vi "LabFrog2.vi"(8 "Simutation":bool, 11 "FROG path":path=path "C:/FROG") -> (0 "error out":errorcluster, 2 "ExpFrog":dbl[][][](array[numeric]), 3 "FROG data":T1[](array[typedef])=[{"Delay increment"=36.8, "Center Wavelength"=809.3, "Frog Error was"=0.0344, "Temporal FWHM"=100.0, "Spectral FWHM"=7.96, "FWHM Time-Bandwidth Product"=0.364, "RMS Time-Bandwidth Product"=0.85}, {"Delay increment"=36.8, "Center Wavelength"=809.3, "Frog Error was"=0.036, "Temporal FWHM"=98.9, "Spectral FWHM"=9.04, "FWHM Time-Bandwidth Product"=0.408, "RMS Time-Bandwidth Product"=0.858}])   [LabVIEW 2018]
doc: "LabFROG \n\nExtract data value from FROG file\n\nAndré Romero - 2022\nandretec@ifsc.usp.br"
uses:
  FROG.ctl
  <vilib>/Utility/file.llb/Read Delimited Spreadsheet (DBL).vi
  <vilib>/regexp/Match Regular Expression.xnode
panel:
  out "index":i32=13
  out "max value (ms)":u32=2
  out "Delay":u32[](array[numeric])=[0, 1, 1, 0, 1, 1, 1, 1, 0, 1, 0, 1, 0, 2, 0, 1, 0, 1, 1, 0, 1, 1, 0, 2, 1, 1, 1, 1, 1, 0, 1, 0, 1, 1, 1, 0, 1, 0, 1]
  out "FROG data":string[][](array[string])=[["32", "32"], ["36.8", "36.8"], ["809.3", "809.3"], ["0.0344", "0.036"], ["100", "98.9"], ["7.96", "9.04"], ["0.364", "0.408"], ["0.85", "0.858"], ["", ""]]
  out "FROG text data":string="Grid characteristics were: 32 points; Delay increment: 36.8 fs; Center Wavelength: 809.3 nm\nFrog Error was: 0.036\nTemporal FWHM: 98.9 fs\nSpectral FWHM: 9.04 nm\nFWHM Time-Bandwidth Product: 0.408\nRMS Time-Bandwidth Product: 0.858\n"
  out "filenames":string[](array[string])=["2022-05-26_10-35-10_ESpectral.dat", "2022-05-26_10-35-10_ETemporal.dat", "2022-05-26_10-35-10_ExpFrog.bmp", "2022-05-26_10-35-10_ExpFrog.dat", "2022-05-26_10-35-10_ExpFrog.jpg", "2022-05-26_10-35-10_Frog.dat", "2022-05-26_10-35-10_RawData.bmp", "2022-05-26_10-35-10_RawData.dat", "2022-05-26_10-35-10_RawData.jpg", "2022-05-26_10-35-10_RawData.png", "2022-05-26_10-35-10_RetrFrog.bmp", "2022-05-26_10-35-10_RetrFrog.dat", "2022-05-26_10-35-10_RetrFrog.jpg", "2022-05-26_10-35-10_screenShot.bmp", "2022-05-26_10-35-10_ss-colorpanel.jpg", "2022-05-26_10-35-10_ss-exper.jpg", "2022-05-26_10-35-10_ss-retrieved.jpg", "2022-05-26_10-35-10_ss-spectral.jpg", "2022-05-26_10-35-10_ss-temporal.jpg", "2022-05-26_10-35-16_ESpectral.dat", "2022-05-26_10-35-16_ETemporal.dat", "2022-05-26_10-35-16_ExpFrog.bmp", "2022-05-26_10-35-16_ExpFrog.dat", "2022-05-26_10-35-16_ExpFrog.jpg", "2022-05-26_10-35-16_Frog.dat", "2022-05-26_10-35-16_RawData.bmp", "2022-05-26_10-35-16_RawData.dat", "2022-05-26_10-35-16_RawData.jpg", "2022-05-26_10-35-16_RawData.png", "2022-05-26_10-35-16_RetrFrog.bmp", "2022-05-26_10-35-16_RetrFrog.dat", "2022-05-26_10-35-16_RetrFrog.jpg", "2022-05-26_10-35-16_screenShot.bmp", "2022-05-26_10-35-16_ss-colorpanel.jpg", "2022-05-26_10-35-16_ss-exper.jpg", "2022-05-26_10-35-16_ss-retrieved.jpg", "2022-05-26_10-35-16_ss-spectral.jpg", "2022-05-26_10-35-16_ss-temporal.jpg", "Thumbs.db"]
  # "[1] Delay increment"
  # "[2] Center Wavelength"
  # "[3] Frog Error was"
  # "[4] Temporal FWHM"
  # "[5] Spectral FWHM"
  # "[6] FWHM Time-Bandwidth Product"
  # "[7] RMS Time-Bandwidth Product"
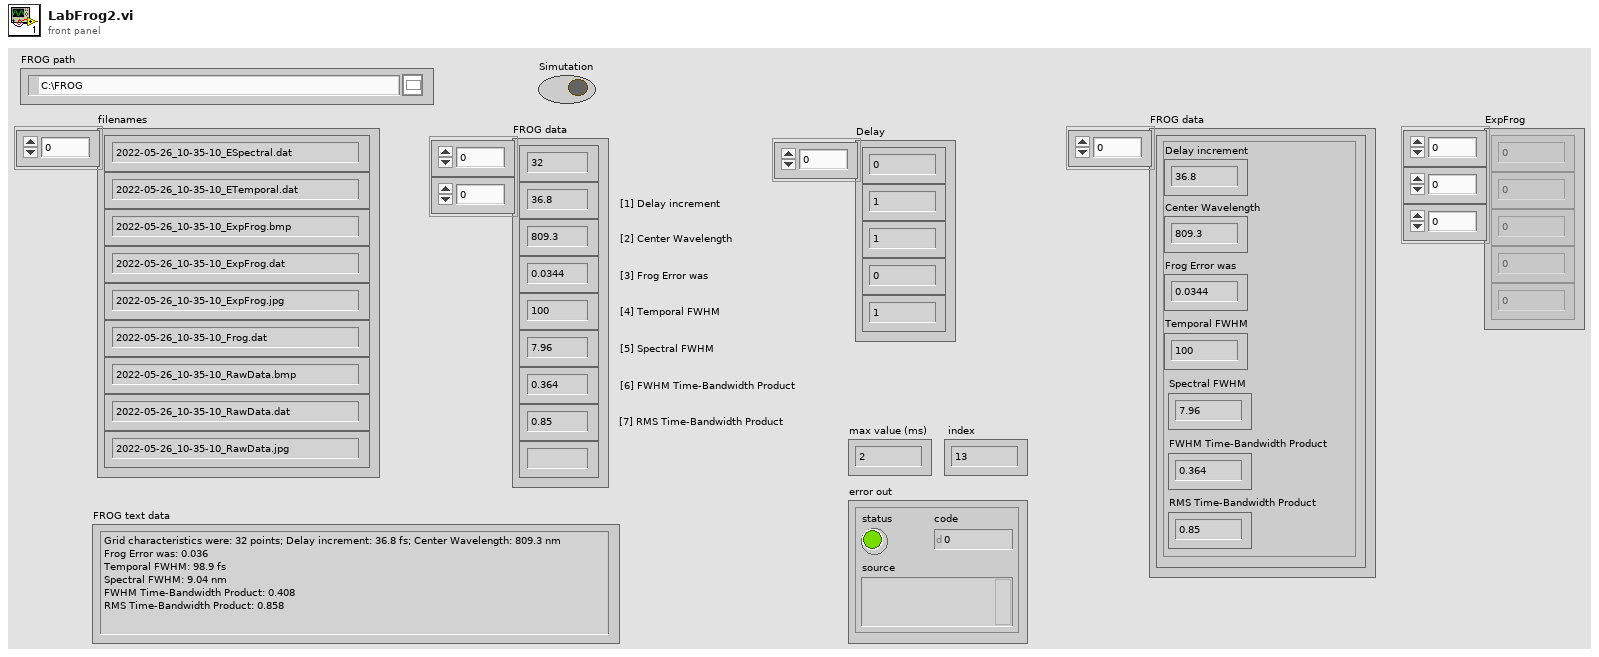
[diagram p1: front panel]
types:
  T1 = typedef "FROG.ctl" = cluster{"Delay increment":dbl, "Center Wavelength":dbl, "Frog Error was":dbl, "Temporal FWHM":dbl, "Spectral FWHM":dbl, "FWHM Time-Bandwidth Product":dbl, "RMS Time-Bandwidth Product":dbl}
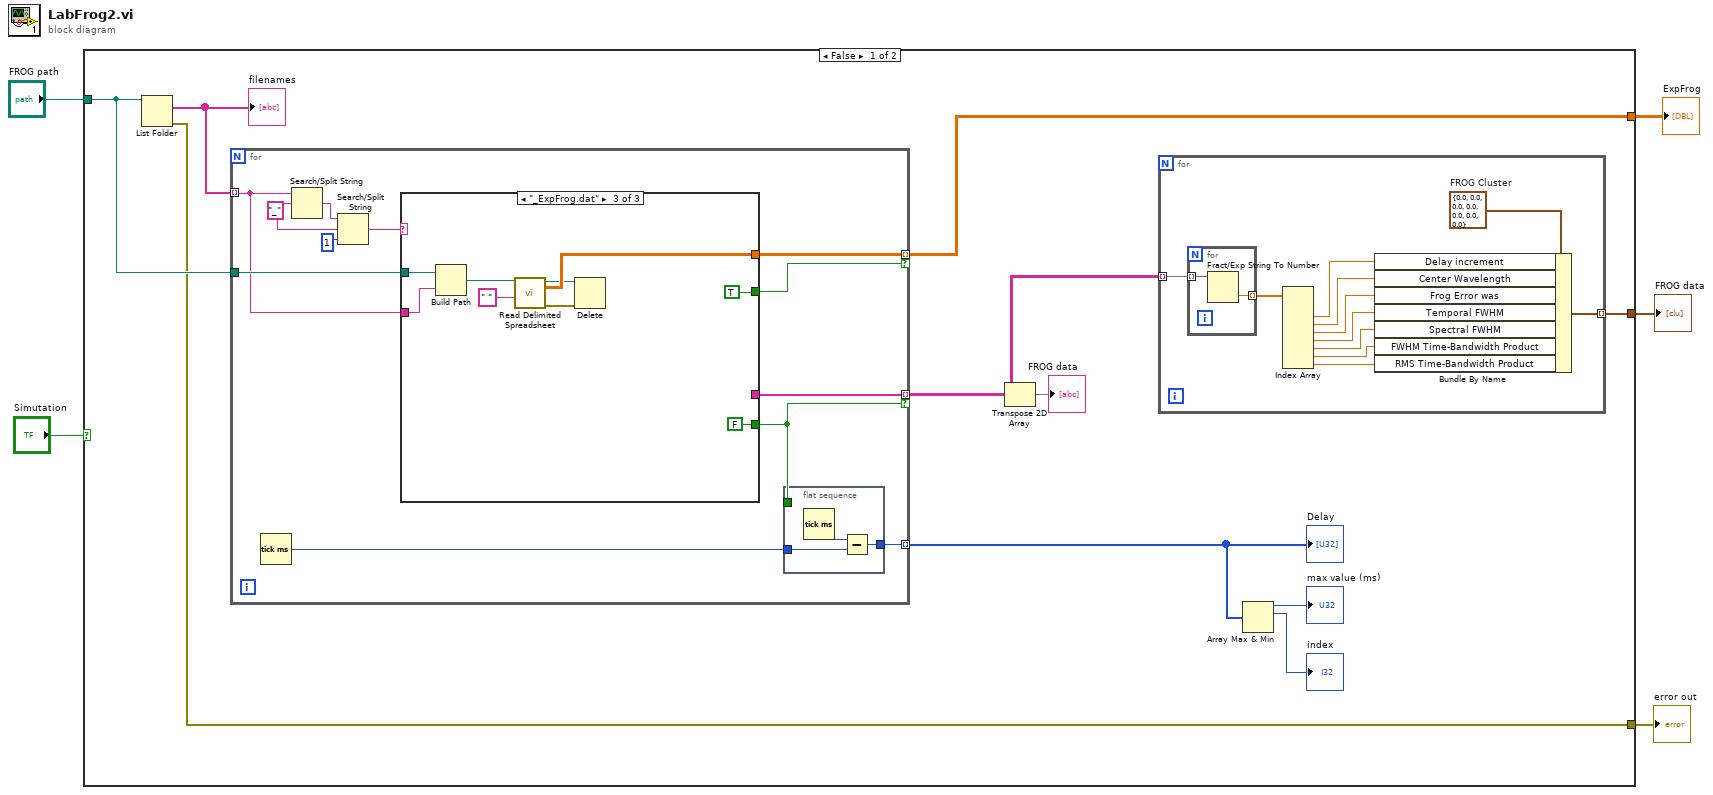
[diagram p0: block diagram]
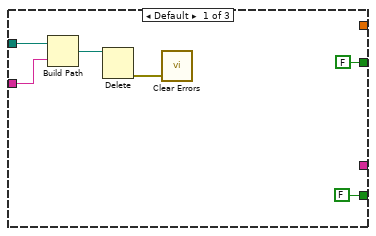
[diagram p2: hidden frame]
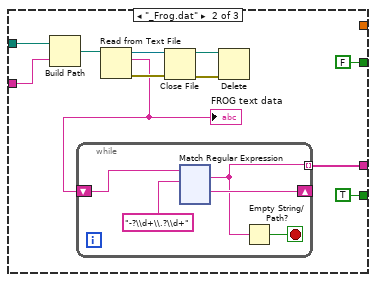
[diagram p3: hidden frame]
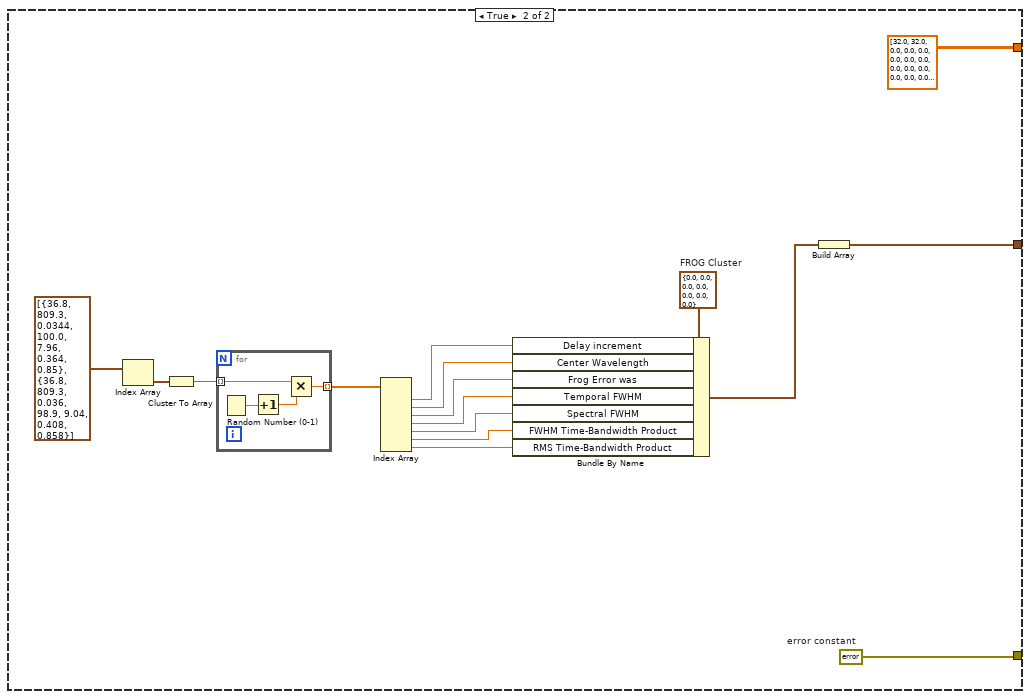
[diagram p4: hidden frame]
diagram:
  n1 = case shown="False" "Simutation" {
    tunnel: "FROG path" -> [w14 _]
    tunnel: [w8 w193] -> w4
    tunnel: [w7 w204] -> w3
    tunnel: [w6 dbl[][][] [[[32.0, 32.0, 0.0, 0.0, 0.0, 0.0, 0.0, 0.0, 0.0, 0.0, 0.0, 0.0, 0.0, 0.0, 0.0, 0.0, 0.0, 0.0, 0.0, 0.0, 0.0, 0.0, 0.0, 0.0, 0.0, 0.0, 0.0, 0.0, 0.0, 0.0, 0.0, 0.0, 0.0], [36.795413510101014, -0.4635609797459772, 404.6559182740907, 0.0, 0.0, 0.0, 0.0, 0.0, 0.0, 0.0, 0.0, 0.0, 0.0, 0.0, 0.0, 0.0, 0.0, 0.0, 0.0, 0.0, 0.0, 0.0, 0.0, 0.0, 0.0, 0.0, 0.0, 0.0, 0.0, 0.0, 0.0, 0.0, 0.0], [0.0, 0.0, 0.0, 0.0, 0.0, 9.383124669467459e-05, 0.0003491815730608666, 0.0, 6.409480248526627e-05, 0.0008864004322777532, 0.000632757752753833, 3.0199503153672837e-05, 7.817832175702415e-05, 2.3518185615836185e-05, 0.0011489734668135715, 0.0019725196109598437, 0.00025194681791796867, 0.0002987599443908123, 0.0, 0.0, 0.0, 0.0, 0.0, 0.0, 0.0, 0.0, 0.0, 0.0009475293472286209, 0.00015758863182998507, 0.000259977394991097, 0.00013913999813479293, 0.0, 0.0], [0.0, 0.0, 0.0, 0.0, 0.0, 0.0002572257670292721, 0.0009402408960831934, 0.0, 0.0001954409853739759, 0.00023678828453734836, 0.0005902309522823148, 0.00012177894336252691, 0.00055494859474722, 0.00027610800338300043, 0.0003477080269209005, 0.00029056585133413134, 0.0003529399393074245, 0.0012830384872731396, 0.0, 0.0, 0.0, 0.0, 0.0, 0.0, 0.0, 0.0, 0.0, 0.001392913654613664, 0.00010596135959795391, 0.0001742656551763975, 0.0006773026116153961, 0.0003886440021940651, 0.0], [0.0, 0.0, 0.0, 0.0, 0.0, 0.000377345962726252, 0.0004029405869775709, 0.0, 0.0, 9.361416048666476e-05, 0.0008945223554809477, 0.0008573902570428489, 0.0, 0.000447542189696726, 0.0008532244402158683, 0.0006819490617583292, 0.0003867968784322788, 4.056579215020924e-05, 0.0, 0.0, 0.0, 0.0, 0.0, 0.0, 0.0, 0.0, 0.0, 0.0004656924543418393, 0.0002521090517443626, 0.0004848829223360913, 0.0004349034287119288, 0.00033515372220337743, 0.0], [0.0, 0.0, 0.0, 0.0, 0.0, 0.00045121456410552127, 0.00010856471709808553, 0.0, 0.0, 0.0, 6.379474984020488e-05, 0.0010420019056774743, 0.0, 0.0, 0.00040334940424008005, 9.94111201803135e-05, 0.0008081914623451595, 0.0, 0.0, 5.6211705004068485e-05, 6.325783570005706e-05, 0.0006788880177273632, 0.0, 0.0, 0.0, 0.0, 0.00022638529816661413, 0.0001110874570151415, 0.000354607755154055, 0.00032502225875306905, 0.0, 0.0, 0.0], [0.0, 0.0, 0.0, 0.0, 0.0, 0.0, 0.0, 0.0, 0.0, 0.0, 0.0002806329836434238, 0.0, 0.0, 0.0, 7.474969661187836e-05, 0.0006404904430431377, 7.987753847568461e-05, 8.120207346022937e-05, 0.0003061135043451707, 0.00017741817635895377, 8.911440590753575e-06, 0.0008925424119134828, 0.00043117805553072623, 0.0, 0.0, 0.0, 0.00014496022249678857, 0.0005679950543386657, 0.0006111202414023585, 0.0, 0.0, 0.0, 0.0], [0.0, 0.0, 0.0, 0.0, 0.0, 0.0, 0.0, 0.0, 0.0, 0.00017038556023809954, 0.0, 0.0, 0.0, 0.00016654966087065502, 0.0012090511684305387, 0.0009117776980965006, 0.0, 0.0005686177179388955, 0.0018097785157693946, 0.0020601457209527465, 0.0029975731058725203, 0.003167796159447548, 0.0025999395403076657, 0.0004747322532108653, 0.00018292693442461093, 0.0014437652073660365, 1.9589287303621454e-05, 0.00026267461778820076, 0.0004162285388923836, 0.0, 0.0, 0.0, 0.0], [0.0, 0.0, 0.0, 0.0, 0.0, 0.0, 0.0, 0.0, 9.717608341963015e-05, 0.0007325250855772218, 2.61880245116324e-05, 0.0, 0.0, 0.0017668869408657276, 0.0012805771728899636, 0.00566275746495714, 0.009738176705029659, 0.010659467302790921, 0.006601452405373148, 0.0020425251324248566, 0.009950506911250899, 0.013708103706214362, 0.005066663155013987, 0.00013838887757807047, 0.00027555670473951993, 0.0009895241219215756, 0.0, 0.0, 0.0006432283896180262, 0.0, 0.0, 0.0, 0.0], [0.0, 0.0, 0.0, 0.0, 0.0, 0.0, 0.0, 0.0, 0.00037099441260831327, 0.0006663020046847149, 0.00012674307708380658, 0.0, 0.0, 0.0014349936740286333, 0.002718389090041099, 0.005270090125313229, 0.017833196032040147, 0.012033867256170932, 0.0004862540056647226, 0.00272106504371272, 0.013189605396490951, 0.008323527128091123, 0.001365785273103551, 0.000886895047861031, 0.0018804612269589273, 0.00032427205120839355, 0.0, 0.0, 0.00033359642370606505, 0.0, 0.0, 0.0, 0.0], [0.0, 0.0, 0.0, 0.0, 0.0, 0.0, 0.0, 0.0, 0.000227719037584713, 0.0009114135456974599, 0.0004873638072713873, 0.000357724533247419, 5.275824555071023e-05, 0.0011832626161023168, 0.0022928311626669697, 0.001086465944123894, 0.0008697144062533685, 0.00037252045994627404, 0.0011415271000469187, 0.0021324914698107374, 0.003843099680410156, 0.0010809594770983754, 0.0019626663730010377, 0.0019268924965370666, 0.000681479939757792, 6.0504991344874336e-05, 0.0, 0.0, 0.0, 0.0, 0.0, 0.0, 0.0], [0.0, 0.0, 0.0, 0.0, 0.0, 0.0, 0.0, 0.0, 0.0, 0.0, 0.002223266039273114, 0.0026636102974912116, 0.0007651509849931216, 0.0009047314743511072, 0.003644349643122779, 0.0010656389715356814, 0.0, 0.0030690863139656603, 0.0068013719208077535, 0.0021224949461464177, 0.0016432460176846078, 0.004765595552209342, 0.018093739546671723, 0.010520899347953654, 0.0018147706501597995, 0.0, 7.653594926508147e-05, 0.0002061651906551166, 0.0, 0.0, 0.0, 0.0, 0.0], [0.0, 0.0, 0.0, 0.0, 0.0, 0.0, 0.00025367829276053816, 0.0, 0.0, 0.0, 0.001381632307706573, 0.004115243944166494, 0.003133443341837566, 0.0008117383907326551, 0.0007620415466116049, 0.004634821365596866, 0.007608824819795769, 0.00915493348972284, 0.006250949527268985, 0.009770781362130063, 0.05037943761555642, 0.06349963620837726, 0.079024262742656, 0.019279214660902967, 0.002215039984900857, 0.00022758785755275097, 0.0012307312962949817, 0.00028772889354737943, 0.0, 0.0, 0.0, 0.0, 0.0], [0.0, 0.0, 0.0, 0.0, 0.0, 0.0, 0.0013544163125227783, 0.0004217071344567472, 0.0002759646526509911, 0.00014997282519262862, 0.00022009615140035983, 0.0014696674767489353, 0.0030642832954310356, 0.0042446477208675955, 0.0053181492498283215, 0.008154366717766077, 0.009928408219650247, 0.03719349957087584, 0.06310666436914894, 0.10053375604005275, 0.1599050504317501, 0.14690116633304237, 0.09941331883378368, 0.01873557410233462, 0.0008249828422071588, 8.755628424353928e-05, 0.0014363252043608737, 0.0011425634367228388, 0.0, 0.0, 0.0, 0.0, 0.0], [0.0, 0.0, 0.0, 0.0, 0.0, 0.00017113003186483946, 0.0027341087488917254, 0.003411575011816168, 0.006829876093085829, 0.004513264011059577, 0.004719758245693675, 0.00597975158317566, 0.010217651411979863, 0.026675265503026752, 0.08143910680272716, 0.14118593063339774, 0.17955897666066467, 0.25321337130604443, 0.25414135646511155, 0.2476732252002294, 0.24758963323776792, 0.1709638639676613, 0.057335479585507984, 0.0062624489204781445, 0.00024063343983997095, 0.001102431619932134, 0.0033780892324134677, 0.002077404885772742, 0.0, 0.0, 0.0, 0.0, 0.0], [0.0, 0.0, 0.0, 0.0, 0.0, 0.0004210492084412745, 0.0038472200691696628, 0.011893761683602547, 0.034696970212626896, 0.03832691258735318, 0.051863486031587705, 0.06189835734134625, 0.07429625615383427, 0.12094528258045883, 0.2178082077833314, 0.43869137975557065, 0.5583413341703908, 0.587703653925067, 0.48871330812850033, 0.27942847952350625, 0.1967231345141605, 0.10783889006587351, 0.024875831705110433, 0.005779697952040987, 0.0064218791996595295, 0.00459929403874266, 0.003918633696610061, 0.0036001781885628887, 0.00047740448623445663, 0.0, 0.0, 0.0, 0.0], [0.0, 0.0, 0.0, 0.0, 0.0, 0.0008092319888367258, 0.007470587624816288, 0.02916426019010017, 0.07876512647197578, 0.12662950349306115, 0.1814859989009447, 0.22529237217192646, 0.25254841293995406, 0.30419449612279786, 0.4087468375728572, 0.5652623943742946, 0.6017588094123656, 0.5852554251753885, 0.3785685997990567, 0.21138838254747278, 0.11516301918375185, 0.09609705833100594, 0.05510272734750322, 0.0430197336738319, 0.021427044350406533, 0.007443677474056787, 0.009121850394608314, 0.005532379102845891, 0.0006725181216096105, 5.482145170470199e-05, 0.0, 0.0, 0.0], [0.0, 0.0, 0.0, 0.0, 0.0, 0.0012959348013429138, 0.01355586016209492, 0.04855345314305047, 0.11653902998548825, 0.21207287968113878, 0.2815149099740793, 0.4084220298951128, 0.5233552591187246, 0.6609255356142588, 0.6363615716319362, 0.7908351978471002, 0.7649887881604941, 0.5106419920092533, 0.45577636954300543, 0.3588453782708846, 0.2582554876054676, 0.25878531239304353, 0.2133494721264744, 0.13916781370776335, 0.07304763907067972, 0.023269115179678963, 0.012832742288956542, 0.007335311445313394, 0.0004982484884586288, 0.0008891612778876077, 0.0, 0.0, 0.0], [0.0, 0.0, 0.0, 0.0, 0.0, 0.000710851841421752, 0.01612357530868892, 0.04723201429012255, 0.11636651424462337, 0.30068754184512514, 0.43524654836793775, 0.5626645267834571, 0.8221465110918468, 1.0, 0.981817354195064, 0.7590179921376713, 0.5715745299908835, 0.5412875208906174, 0.5484306548644949, 0.5332664114017821, 0.5041480899733091, 0.4686844141783367, 0.3666564265863091, 0.22290713137333767, 0.1019741981140139, 0.030822341340646996, 0.01628987651090177, 0.006064125855667253, 0.0020724877445948303, 0.0012330879780934694, 0.00013459023128587096, 0.0, 0.0], [0.0, 0.0, 0.0, 0.0, 0.0, 0.001171662808504237, 0.013048585365156419, 0.04702185972909596, 0.10506858675145546, 0.232727521284574, 0.3135434046833827, 0.4173680444367505, 0.6619723792582326, 0.8380458569261603, 0.7934498127878032, 0.6836975020173057, 0.6592417581625181, 0.6233905254300568, 0.6215497507808431, 0.5561423003975796, 0.543719489211694, 0.4575460552229224, 0.4385914377129764, 0.23915532147943364, 0.13970584522864635, 0.08962561661419381, 0.026706676351902277, 0.011980224595163081, 0.005432340827235229, 0.0004967427029115903, 0.00010243907811546027, 0.0, 0.0], [0.0, 0.0, 0.0, 0.0, 0.0, 0.0, 0.007155519442263225, 0.024667471518022375, 0.07941529683523231, 0.13535871701290708, 0.21554242668936094, 0.3234262319282746, 0.37189190698345925, 0.37062802887194524, 0.35166429071451827, 0.28620951247051907, 0.2541541813376154, 0.2277282996487241, 0.26551743257486243, 0.2904185641893251, 0.32278092320610596, 0.34345416291161024, 0.32186130659916645, 0.2089852481796307, 0.11669164654423372, 0.07578041735272707, 0.025758842142133285, 0.010950760422172759, 0.006603168370813867, 0.0003160407305213402, 0.0, 0.0, 0.0], [0.0, 0.0, 0.0, 0.0, 0.0, 0.0, 0.0018389346669078202, 0.01068181774931775, 0.044672791002046165, 0.08443702726274892, 0.10637876629394383, 0.1661924473750489, 0.1877157204826251, 0.18873523604620174, 0.18961878300212726, 0.21989776056136506, 0.2340622781075487, 0.20077588045195865, 0.12112671093952265, 0.07618690086309017, 0.09163738721552259, 0.09670627621931192, 0.10819869754849543, 0.10644001582855768, 0.062471361373287314, 0.03187656282306997, 0.01606767268441069, 0.00778944820518461, 0.003883975297185835, 0.0003461839890780148, 0.0, 0.0, 0.0], [0.0, 0.0, 0.0, 0.0, 0.0, 0.0, 0.0015887345755627265, 0.007737844485060771, 0.013464399242779031, 0.028227675865846985, 0.029081917327884673, 0.03567202771329378, 0.02746027827273163, 0.013395151113464624, 0.0342532575354353, 0.13380737959215033, 0.25551813658471895, 0.3054897813243066, 0.2154599733958421, 0.10698255024014357, 0.03263213078464283, 0.012997539964106613, 0.01361947254871387, 0.020275153819555736, 0.018193218912982725, 0.010172178951428811, 0.006873092255059616, 0.003599736762453299, 0.0022078217606024356, 0.00044364187484989873, 0.0, 0.0, 0.0], [0.0, 0.0, 0.0, 0.0, 0.0, 0.0, 0.0, 0.0015990490761984245, 0.0035652071148236054, 0.001647920534366952, 0.0008168870135220761, 0.0006293335014487618, 0.00016673798972069388, 0.00014245942089899467, 0.01168045587905908, 0.05075246893855485, 0.12246295626832762, 0.1713716313555505, 0.15849022665404863, 0.1408376526131936, 0.10794377499596176, 0.04208348332322521, 0.0052420232631775875, 0.00099529930692507, 0.0035419718515921294, 0.004406594750157155, 0.0027911422763838064, 0.0013553046466565654, 0.0015081851164192956, 0.00030095605592398204, 0.0, 0.0, 0.0], [0.0, 0.0, 0.0, 0.0, 0.0, 0.0, 0.0, 0.0, 0.0004449848649267463, 0.0, 0.00043363824239867315, 0.0025343513092985696, 0.0006296677604763472, 0.0, 0.0020342410331099844, 0.004871187798428841, 0.007652884345180917, 0.017089227223144696, 0.047197455072608384, 0.09421655969106786, 0.12584582666056615, 0.110747084849056, 0.05562123692430584, 0.011115350241111911, 0.0010592547071157348, 0.0010263780652249165, 0.0011824021629660154, 0.0021254762094508627, 0.0006663081538130516, 5.005730049699086e-05, 0.0, 0.0, 0.0], [0.0, 0.0, 0.0, 0.0, 0.0, 0.0, 0.0, 0.0, 0.0, 0.0, 0.00025762479163655294, 0.004454175966748375, 0.0, 0.0, 0.0, 0.0016755789128175917, 0.0008917846936307861, 0.0012058782976116914, 0.003409216926231585, 0.012891087966765906, 0.049990143425970024, 0.08930427284184123, 0.06586143840835912, 0.018785633540244213, 0.003431703179169783, 0.0008796393747060783, 0.0007745742429200142, 0.0013875934762228558, 0.0007998870048600161, 0.0007885307695308276, 0.0, 0.0, 0.0], [0.0, 0.0, 0.0, 0.0, 0.0, 0.0, 0.0, 0.0, 0.0, 0.0, 0.0, 0.0011954680756742768, 0.0, 0.0, 0.0, 0.0, 0.0, 0.0005549871178185541, 0.0006094780879968187, 0.00047296605747190127, 0.00602920639800985, 0.01533784232228132, 0.02544227193283859, 0.009836078443824394, 0.0023247584381713626, 0.00033840977261154236, 0.0002417602927826612, 0.00025910450664819894, 0.0011679980459357007, 0.0005285606896082035, 0.0, 0.0, 0.0], [0.0, 0.0, 0.0, 0.0, 0.0, 0.0, 0.0, 0.0, 0.0, 0.0, 0.0, 0.0, 0.0, 0.0, 0.0, 4.1433283512810445e-05, 0.00024667904042756925, 0.00025401989028475707, 0.0004255050415615293, 0.0012243883214507019, 0.0002883226969153251, 0.00045199597808435424, 0.003606949514337155, 0.004287380972710013, 0.00391903261485719, 0.002399932898888551, 0.0, 0.0, 0.0004591872517728951, 0.0, 0.0, 0.0, 0.0], [0.0, 0.0, 0.0, 0.0, 0.0, 0.0, 0.0, 0.0, 0.0, 0.0, 0.0, 0.0, 0.0, 0.0, 0.0, 0.0013007560314556897, 0.01208804832035635, 0.002996915387723811, 0.002013604838186929, 0.0012566259468198893, 0.0035850652688129295, 0.002181805707520993, 0.00013333811206203412, 0.0007640580338572978, 0.0016233072898789135, 0.0016778659711971736, 0.0, 0.0, 0.0, 0.0, 0.0, 0.0, 0.0], [0.0, 0.0, 0.0, 0.0, 0.0, 0.0, 0.0, 0.0, 0.0, 0.0, 0.0, 0.0, 0.0, 0.0, 0.0, 0.0, 0.004088273525725404, 0.0021996946174284463, 0.0030700917995289123, 0.00697916577463041, 0.00715279932266826, 0.007511243459095975, 0.002416106399597258, 0.0, 0.0003175276722806536, 0.00029029675574205065, 0.0, 0.0, 0.0, 0.0, 0.0, 0.0, 0.0], [0.0, 0.0, 0.0, 0.0, 0.0, 0.0, 0.0, 0.0, 0.0, 0.0, 0.0, 0.0, 0.0, 0.0, 0.0, 0.0, 0.0, 6.703429279446747e-05, 0.00019341178572042958, 0.0007005173521887295, 0.0025464475008170283, 0.0038933551004845025, 0.002587305476707822, 0.0010831489393612864, 0.000433531246577368, 0.0, 0.0, 0.0, 0.0, 0.0, 0.0, 0.0, 0.0], [0.0, 0.0, 0.0, 0.0, 0.0, 0.0, 0.0, 0.0, 0.0, 0.0, 0.0, 0.0, 0.0, 0.0, 0.0, 0.0, 0.0, 0.0, 0.0, 0.0, 0.00022675355474310408, 0.0004736576726994118, 0.0004633021595951355, 0.0002985762767068883, 0.0001247322336969134, 0.0, 0.0, 0.0, 0.0, 0.0, 0.0, 0.0, 0.0], [0.0, 0.0, 0.0, 0.0, 0.0, 0.0, 0.0, 0.0, 0.0, 0.0, 0.0, 0.0, 0.0, 0.0, 0.0, 0.0, 0.0, 0.0, 0.0, 0.0, 0.0, 0.0, 0.0, 0.0, 0.0, 0.0, 0.0, 0.0, 0.0, 0.0, 0.0, 0.0, 0.0], [0.0, 0.0, 0.0, 0.0, 0.0, 0.0, 0.0, 0.0, 0.0, 0.0, 0.0, 0.0, 0.0, 0.0, 0.0, 0.0, 0.0, 0.0, 0.0, 0.0, 0.0, 0.0, 0.0, 0.0, 0.0, 0.0, 0.0, 0.0, 0.0, 0.0, 0.0, 0.0, 0.0]], [[32.0, 32.0, 0.0, 0.0, 0.0, 0.0, 0.0, 0.0, 0.0, 0.0, 0.0, 0.0, 0.0, 0.0, 0.0, 0.0, 0.0, 0.0, 0.0, 0.0, 0.0, 0.0, 0.0, 0.0, 0.0, 0.0, 0.0, 0.0, 0.0, 0.0, 0.0, 0.0, 0.0], [36.795413510101014, -0.4635609797459772, 404.6559182740907, 0.0, 0.0, 0.0, 0.0, 0.0, 0.0, 0.0, 0.0, 0.0, 0.0, 0.0, 0.0, 0.0, 0.0, 0.0, 0.0, 0.0, 0.0, 0.0, 0.0, 0.0, 0.0, 0.0, 0.0, 0.0, 0.0, 0.0, 0.0, 0.0, 0.0], [0.0, 0.0, 0.0, 0.0, 0.0, 0.0, 0.0, 0.0, 0.0, 0.0, 0.0, 0.0, 0.0, 0.0, 0.0, 0.0, 0.0, 0.0, 0.0, 0.0, 0.0, 0.0, 0.0, 0.0, 0.0, 0.0, 0.0, 0.0, 0.0, 0.0, 0.0, 0.0, 0.0], [0.0, 0.0, 0.0, 0.0, 0.0, 0.0, 0.0, 0.0, 0.0, 0.0, 0.0, 0.0, 0.0, 0.0, 0.0, 0.0, 0.0, 0.0, 0.0, 0.0, 0.0, 0.0, 0.0, 0.0, 0.0, 0.0, 0.0, 0.0, 0.0, 0.0, 0.0, 0.0, 0.0], [0.0, 0.0, 0.0, 0.0, 0.0, 0.0, 0.0, 0.0, 0.0, 0.0, 0.0, 0.0, 0.0, 0.0, 0.0, 0.0, 0.0, 0.0, 0.0, 0.0, 0.0, 0.0, 0.0, 0.0, 0.0, 0.0, 0.0, 0.0, 0.0, 0.0, 0.0, 0.0, 0.0], [0.0, 0.0, 0.0, 0.0, 0.0, 0.0, 0.0, 0.0, 0.0, 0.0, 0.0, 0.0, 0.0, 0.0, 0.0, 0.0, 0.0, 0.0, 0.0, 0.0, 0.0, 0.0, 0.0, 0.0, 0.0, 0.0, 0.0, 0.0, 0.0, 0.0, 0.0, 0.0, 0.0], [0.0, 0.0, 0.0, 0.0, 0.0, 0.0, 0.0, 0.0, 0.0, 0.0, 0.0, 0.0, 0.0, 0.0, 0.0, 0.0, 0.0, 0.0, 0.0, 0.0, 0.0, 0.0002982319878017142, 0.0, 0.0, 0.0, 0.0, 0.0, 0.0, 0.0, 0.0, 0.0, 0.0, 0.0], [0.0, 0.0, 0.0, 0.0, 0.0, 0.0, 0.0, 0.0, 0.0, 0.0, 0.0, 0.0, 0.0, 0.0, 0.0, 0.0001878612062683148, 1.4224128374984825e-05, 0.0004340066103293415, 0.002393988006969019, 0.0009560952344966215, 0.0010191697833653703, 0.0023976584306842704, 0.002136922673905889, 0.0, 0.0, 0.0, 0.0, 0.0, 0.0, 0.0, 0.0, 0.0, 0.0], [0.0, 0.0, 0.0, 0.0, 0.0, 0.0, 0.0, 0.0, 0.0, 0.0, 0.0, 0.0, 0.0, 0.0, 0.00011038146753699227, 0.005656253781830486, 0.009807817695364835, 0.012434705591390418, 0.008326470866208992, 0.0013601316486306424, 0.010298936111138505, 0.012226358115841756, 0.006400158434440107, 0.00045348002692052264, 0.0, 0.0, 0.0, 0.0, 0.0, 0.0, 0.0, 0.0, 0.0], [0.0, 0.0, 0.0, 0.0, 0.0, 0.0, 0.0, 0.0, 0.0, 0.0, 0.0, 0.0, 0.0, 0.0, 0.001561409609642338, 0.004523120789769258, 0.0174012287292024, 0.010794787528224726, 0.0005766630248207759, 0.0018409715711076166, 0.016096594078239063, 0.007502742263145624, 0.0017873163777441562, 0.00215572969207354, 0.002012088453040024, 0.0, 0.0, 0.0, 0.0, 0.0, 0.0, 0.0, 0.0], [0.0, 0.0, 0.0, 0.0, 0.0, 0.0, 0.0, 0.0, 0.0, 0.0, 0.0, 0.0005809166733911795, 9.680881451035746e-06, 0.0, 0.00013273216308756143, 0.0007279166555593684, 0.0, 0.00035405816218315734, 0.0, 0.0018309321919789548, 0.0025709155014665124, 0.0010234857560877835, 0.002252720764724932, 0.003627785226639823, 0.0007628846408034042, 0.0, 0.0, 0.0, 0.0, 0.0, 0.0, 0.0, 0.0], [0.0, 0.0, 0.0, 0.0, 0.0, 0.0, 0.0, 0.0, 0.0, 0.0, 0.00028103283528680263, 0.0037152055279272757, 0.00021425967213339897, 0.0, 0.0018775731069536352, 0.0003587509184572551, 0.0, 0.002362755611362491, 0.00927450986169844, 0.0023554272828160147, 0.002114430273777235, 0.007915886083423617, 0.021568597870283833, 0.013981267953223039, 0.002366451897926433, 0.0, 0.0, 0.0, 0.0, 0.0, 0.0, 0.0, 0.0], [0.0, 0.0, 0.0, 0.0, 0.0, 0.0, 0.0, 0.0, 0.0, 0.0, 0.0011377686987944836, 0.0043674147011671365, 0.0013614224970071801, 4.1719067459375507e-05, 9.30028838421002e-06, 0.0023868951236835695, 0.007023616871548888, 0.010850791476718868, 0.007331778951124423, 0.010315243596059237, 0.05477987173165404, 0.07110332170201876, 0.08030611668962213, 0.026250372158863226, 0.000844036687502042, 0.0, 0.0, 0.0, 0.0, 0.0, 0.0, 0.0, 0.0], [0.0, 0.0, 0.0, 0.0, 0.0, 0.0, 0.0003765690085485011, 0.0005862163985229224, 0.0009935880097798437, 0.0, 0.0, 0.0022165532504815895, 0.0029706599190998688, 0.002113191836517556, 0.005663247828509422, 0.006562849924606898, 0.014933146070690025, 0.040646432717544576, 0.06698133805445054, 0.10477256692993143, 0.1647282316979872, 0.14850759293979388, 0.10210181699143174, 0.023325011534717683, 0.0, 0.0, 0.0006909794441389231, 0.000624520126904273, 0.0, 0.0, 0.0, 0.0, 0.0], [0.0, 0.0, 0.0, 0.0, 0.0, 0.0, 0.001378234915312134, 0.0041294488519760105, 0.008428268330931528, 0.004375177871996265, 0.006555542607647751, 0.006475233053480385, 0.010994790887748285, 0.02691515481112869, 0.09277822897076075, 0.14744939435295148, 0.18966028518253247, 0.26273949967812466, 0.26057334279565614, 0.25192565258060456, 0.24727728880435892, 0.1672164935227077, 0.05788938719269681, 0.006190926519337974, 0.0, 0.0013143737500521332, 0.0025185176004983334, 0.0011169815465052267, 0.0, 0.0, 0.0, 0.0, 0.0], [0.0, 0.0, 0.0, 0.0, 0.0, 0.0002251755795486918, 0.0030012681978811794, 0.01220617426209216, 0.033451982654730865, 0.04155807329829025, 0.06032499675055803, 0.06470141200709872, 0.07834753433931108, 0.12913567752810534, 0.23211493184017964, 0.4577295628990756, 0.5696900378017434, 0.6048655079046267, 0.4954295520813375, 0.2800765063320248, 0.1968573254726476, 0.10678616236066127, 0.027865076891887317, 0.003196650307428739, 0.005504435871130102, 0.0029460308983497627, 0.0055376790799639905, 0.0026527685049465895, 0.0, 0.0, 0.0, 0.0, 0.0], [0.0, 0.0, 0.0, 0.0, 0.0, 0.0007010238088434504, 0.006721057605331844, 0.027811389369675688, 0.08216174314110657, 0.13428290285669367, 0.18564253934719768, 0.22360704767861805, 0.25427703032389515, 0.31392492318759335, 0.4165005542507313, 0.5711690600656787, 0.6164681256269003, 0.5954784125509031, 0.37789481959023513, 0.21888748641741745, 0.11202935562676448, 0.09999054911772351, 0.05806026049465249, 0.04470630474168452, 0.024001366707243402, 0.005955851650703747, 0.009332249519769322, 0.0057582759325952035, 9.694345224408757e-05, 0.0, 0.0, 0.0, 0.0], [0.0, 0.0, 0.0, 0.0, 0.0, 0.0005368624622113731, 0.011343006484288277, 0.046610155993410916, 0.12190290242609911, 0.22292329744792488, 0.2913399488303097, 0.41130291294618415, 0.53115111638282, 0.6588623294022311, 0.6358031675347707, 0.7908373597653081, 0.7746486129897366, 0.5094830216740359, 0.4538846987150514, 0.3600752665992875, 0.2648833019786846, 0.26145505311615763, 0.22290297449973787, 0.14150805998539087, 0.07276532040225453, 0.02471965288653826, 0.01592769258109848, 0.006178719608461857, 0.001248444531290498, 0.0, 0.0, 0.0, 0.0], [0.0, 0.0, 0.0, 0.0, 0.0, 1.9609064397576527e-05, 0.014277819588327953, 0.046068613691219625, 0.11292216979531347, 0.3083489852097657, 0.4440573348909483, 0.5654342277725061, 0.8235278770111891, 1.0, 0.9688614712216062, 0.7427498473657047, 0.5599836007886722, 0.5383220854352196, 0.554895915886854, 0.5471944286759057, 0.508627423958084, 0.47782033690622977, 0.37833224685233957, 0.22720214315486498, 0.10665074236976194, 0.03662245065375156, 0.019164448086862747, 0.004923721143254672, 0.0007773227929689036, 0.0, 0.0, 0.0, 0.0], [0.0, 0.0, 0.0, 0.0, 0.0, 0.00036508731311658886, 0.010959996009964031, 0.044473494403692616, 0.10341555143293445, 0.2307162842667621, 0.3111095713171326, 0.4183831939279572, 0.6585218470858754, 0.8310255169161711, 0.7771606961801757, 0.6691541707546823, 0.6442351912708392, 0.6139861077385969, 0.6369843414106354, 0.5713168478960252, 0.5489148096564311, 0.4724080375916645, 0.4464241623151682, 0.24761968106680024, 0.14173403142814053, 0.08811443107769494, 0.02499096231396023, 0.011817240927341212, 0.0026642505358419554, 0.0, 0.0, 0.0, 0.0], [0.0, 0.0, 0.0, 0.0, 0.0, 0.0005799589148534439, 0.005034139542607277, 0.02106536285411135, 0.07847302822671147, 0.14142278567738437, 0.2105572161363529, 0.3203175567777369, 0.36504873938615223, 0.36374815769021895, 0.34054776971621437, 0.2864190710400675, 0.24622058247481982, 0.22045105796638362, 0.26080354425054164, 0.2987546763623469, 0.3369433600291245, 0.3637916387695826, 0.3360719336296095, 0.2125668149318466, 0.12204302991395496, 0.07548140878265598, 0.021009247905152777, 0.012980662867313142, 0.0029688913961298112, 0.0, 0.0, 0.0, 0.0], [0.0, 0.0, 0.0, 0.0, 0.0, 0.0, 0.0012840456130784183, 0.011692440696309403, 0.039606566941833066, 0.08447965565908364, 0.10473410095551801, 0.16597234605559272, 0.1822155108295753, 0.18387562971680008, 0.18983801964624913, 0.21427814312771004, 0.23874273115796715, 0.19261732963877506, 0.11896906119257596, 0.0785273484447369, 0.10087748797373473, 0.10452117679026868, 0.12283358145986133, 0.11039096705355146, 0.07108419402332142, 0.033597698837634325, 0.011790443049536138, 0.009795566560944274, 0.0009379162333568367, 0.0, 0.0, 0.0, 0.0], [0.0, 0.0, 0.0, 0.0, 0.0, 0.0, 0.0011241600865715526, 0.006008187195139522, 0.012745195156792542, 0.025637822270462778, 0.02821036262850858, 0.030835450822677215, 0.028093008495337003, 0.012079132497305927, 0.02802379057217387, 0.13430407717339995, 0.26120754294754994, 0.31504051892176216, 0.21770705261529902, 0.10891775508629684, 0.0369949898508197, 0.011560105752958579, 0.017567799599541467, 0.024270619583228285, 0.02255190448744352, 0.010704263887534142, 0.005015331665318231, 0.004378346243183401, 0.0003749962422274412, 0.0, 0.0, 0.0, 0.0], [0.0, 0.0, 0.0, 0.0, 0.0, 0.0, 0.0001718451543890687, 0.0014774628392721612, 0.0018669835251368559, 0.000687321162468302, 0.0005099009629315026, 0.0, 0.0, 7.15817760244864e-05, 0.012521942298218678, 0.04541536034067672, 0.1253856645845933, 0.17342993123332065, 0.16772703454686366, 0.14215715903852472, 0.10927184505378457, 0.0397921483492689, 0.006231501256714829, 0.001535967400083123, 0.0034895296748848957, 0.0037284587199560215, 0.0015027009134503703, 0.00168305104614656, 0.0018899355663259967, 0.0, 0.0, 0.0, 0.0], [0.0, 0.0, 0.0, 0.0, 0.0, 0.0, 0.0, 0.0, 0.0, 0.0, 0.0003774603297271909, 0.0, 0.0, 0.0, 0.0006337775270863049, 0.005517084464503666, 0.00539748289110835, 0.019250782695943318, 0.05447881905349352, 0.09444342152177672, 0.129675008714899, 0.11441004257826398, 0.05697048476945565, 0.01256352507866394, 0.00027458148378548046, 0.0008259540184244277, 0.0003200493177929992, 0.000834533658624473, 0.0011171495723192877, 0.0, 0.0, 0.0, 0.0], [0.0, 0.0, 0.0, 0.0, 0.0, 0.0, 0.0, 0.0, 0.0, 0.0, 0.0, 0.0, 0.0, 0.0, 0.0, 0.0005415701366934091, 0.0015746868434241685, 0.0008234872568136591, 0.003285143498448067, 0.015592126288097044, 0.05190218266320903, 0.09519294127704479, 0.07178927428140816, 0.017356773468227126, 0.0010827833340881067, 0.0, 4.2405013466050355e-05, 0.00013719642851711341, 0.0, 0.0, 0.0, 0.0, 0.0], [0.0, 0.0, 0.0, 0.0, 0.0, 0.0, 0.0, 0.0, 0.0, 0.0, 0.0, 0.0, 0.0, 0.0, 0.0, 0.0, 0.0, 0.0007091766677935631, 0.0012018074395855874, 0.0007465108940436679, 0.005904578300059139, 0.01784750836105234, 0.03389768636044688, 0.009393292817004994, 0.0008888146133953778, 0.0, 0.0, 0.0, 0.0, 0.0, 0.0, 0.0, 0.0], [0.0, 0.0, 0.0, 0.0, 0.0, 0.0, 0.0, 0.0, 0.0, 0.0, 0.0, 0.0, 0.0, 0.0, 0.0, 0.0, 0.0, 2.3796216964824254e-05, 0.0005088468031903008, 0.00018053527091219752, 0.0008706691989015834, 0.0006317436770593312, 0.004830313512156658, 0.006497570458709682, 0.003471733571604518, 0.0, 0.0, 0.0, 0.0, 0.0, 0.0, 0.0, 0.0], [0.0, 0.0, 0.0, 0.0, 0.0, 0.0, 0.0, 0.0, 0.0, 0.0, 0.0, 0.0, 0.0, 0.0, 0.0, 0.0, 0.0, 0.002660054380612277, 3.0035896503641105e-05, 1.9845470467148055e-05, 0.0009379053341404909, 0.003364670885195902, 0.0, 0.001473019844083747, 0.002180215963182838, 0.0, 0.0, 0.0, 0.0, 0.0, 0.0, 0.0, 0.0], [0.0, 0.0, 0.0, 0.0, 0.0, 0.0, 0.0, 0.0, 0.0, 0.0, 0.0, 0.0, 0.0, 0.0, 0.0, 0.0, 0.0, 0.0013907831885240605, 0.0, 0.0, 0.0029030436229565623, 0.010377648301216333, 0.0015788053622575974, 0.0, 0.0003584147134477203, 0.0, 0.0, 0.0, 0.0, 0.0, 0.0, 0.0, 0.0], [0.0, 0.0, 0.0, 0.0, 0.0, 0.0, 0.0, 0.0, 0.0, 0.0, 0.0, 0.0, 0.0, 0.0, 0.0, 0.0, 0.0, 4.438093787477861e-05, 0.0, 0.0, 0.00042268955002287026, 0.0038969726812830823, 0.0003899704287799233, 0.0, 0.0, 0.0, 0.0, 0.0, 0.0, 0.0, 0.0, 0.0, 0.0], [0.0, 0.0, 0.0, 0.0, 0.0, 0.0, 0.0, 0.0, 0.0, 0.0, 0.0, 0.0, 0.0, 0.0, 0.0, 0.0, 0.0, 0.0, 0.0, 0.0, 0.0, 0.000390817005528973, 0.0, 0.0, 0.0, 0.0, 0.0, 0.0, 0.0, 0.0, 0.0, 0.0, 0.0], [0.0, 0.0, 0.0, 0.0, 0.0, 0.0, 0.0, 0.0, 0.0, 0.0, 0.0, 0.0, 0.0, 0.0, 0.0, 0.0, 0.0, 0.0, 0.0, 0.0, 0.0, 0.0, 0.0, 0.0, 0.0, 0.0, 0.0, 0.0, 0.0, 0.0, 0.0, 0.0, 0.0], [0.0, 0.0, 0.0, 0.0, 0.0, 0.0, 0.0, 0.0, 0.0, 0.0, 0.0, 0.0, 0.0, 0.0, 0.0, 0.0, 0.0, 0.0, 0.0, 0.0, 0.0, 0.0, 0.0, 0.0, 0.0, 0.0, 0.0, 0.0, 0.0, 0.0, 0.0, 0.0, 0.0]]] ("all rows 2")] -> w1
    frame False {
      n2 = List Folder(path=w14) -> (filenames=w15:string[], error out=w7:errorcluster)  [unwired: 3 in, 2 out]
      "filenames" <- w15
      n3 = for {
        tunnel: w15 -> [w31] mode=indexing
        tunnel: w14 -> [w40]
        tunnel: [w36] -> w9 mode=indexing if=w39
        tunnel: [w37] -> w12 mode=indexing
        tunnel: [w30] -> w6 mode=indexing if=w29
        w34 = "_" ("search string/char (-)")
        n4 = Tick Count (ms)() -> (millisecond timer value=w38:u32)
        n5 = Search/Split String(string=w31, search string/char (-)=w34) -> (match + rest of string=w35:string)  [unwired: 1 in, 2 out]
        n6 = Search/Split String(string=w35, search string/char (-)=w34, offset (0)=1) -> (match + rest of string=w32:string)  [unwired: 2 out]
        n7 = case shown="\"_ExpFrog.dat\"" w32 {
          tunnel: w31 -> [w45 w59 w186]
          tunnel: w40 -> [w48 w60 w187]
          tunnel: [_ w57 _] -> w36
          tunnel: [FALSE TRUE FALSE] -> w39
          tunnel: [_ _ w183] -> w30
          tunnel: [FALSE FALSE TRUE] -> w29
          frame Default {
            n8 = Build Path(base path=w48, name or relative path=w45) -> (appended path=w47:path)
            n9 = Delete(path (use dialog)=w47) -> (error out=w46:errorcluster)  [unwired: 4 in, 2 out]
            n10 = call <vilib>:"Clear Errors.vi"("error in (no error)"=w46) -> ()  [unwired: 5 in, 2 out]
          }
          frame "_Frog.dat" {
            n11 = Build Path(base path=w60, name or relative path=w59) -> (appended path=w58:path)
            n12 = Read from Text File(file (use dialog)=w58) -> (refnum out=w56:refnum<file>, text=w54:string, error out=w55:errorcluster)  [unwired: 3 in, 1 out]
            "FROG text data" <- w54
            n13 = while {
              shift-right: [w63] -> _
              shift-left: w54 -> [w65]
              tunnel: [w62] -> w57 mode=indexing
              stop <- w61 stop-if-true
              n14 = xnode "Match Regular Expression"("input string"=w65, "regular expression"="-?\\d+\\.?\\d+") -> ("whole match"=w62:string, "after match"=w63:string)  [unwired: 4 in, 3 out]
              n15 = Empty String/Path?(string/path=w62) -> (empty?=w61:bool)
            }
            n16 = Close File(refnum=w56, error in=w55) -> (path=w51:path, error out=w52:errorcluster)
            n17 = Delete(path (use dialog)=w51, error in=w52) -> ()  [unwired: 3 in, 3 out]
          }
          frame "_ExpFrog.dat" {
            n18 = Build Path(base path=w187, name or relative path=w186) -> (appended path=w185:path)
            n19 = call-poly <vilib>:"Read Delimited Spreadsheet.vi"("file path (dialog if empty)"=w185, "delimiter (\\t)"=" " ("delimiter (\\t)")) -> ("new file path (Not A Path if cancelled)"=w182:path, "all rows"=w183:dbl[][], "error out"=w181:errorcluster)  [unwired: 8 in, 3 out]
            n20 = Delete(path (use dialog)=w182, error in=w181) -> ()  [unwired: 3 in, 3 out]
          }
        }
        n21 = flat-sequence {
          tunnel: w39 -> [_]
          tunnel: w38 -> [w42]
          tunnel: [w41] -> w37
          frame #0 {
            n22 = Tick Count (ms)() -> (millisecond timer value=w43:u32)
            n23 = Subtract(x=w43, y=w42) -> (x-y=w41:u32)
          }
        }
      }
      "Delay" <- w12
      n24 = Transpose 2D Array(2D array=w9) -> (transposed array=→"FROG data":string[][])
      n25 = for {
        tunnel: w9 -> [w26] mode=indexing
        tunnel: [w16] -> w8 mode=indexing
        w24 = T1 {"Delay increment"=0.0, "Center Wavelength"=0.0, "Frog Error was"=0.0, "Temporal FWHM"=0.0, "Spectral FWHM"=0.0, "FWHM Time-Bandwidth Product"=0.0, "RMS Time-Bandwidth Product"=0.0}  # FROG Cluster
        n26 = for {
          tunnel: w26 -> [w28] mode=indexing
          tunnel: [w27] -> w25 mode=indexing
          n27 = Fract/Exp String To Number(string=w28) -> (number=w27:dbl)  [unwired: 3 in, 1 out]
        }
        n28 = Index Array(array=w25) -> (element #2=w17:dbl, element #3=w18:dbl, element #4=w19:dbl, element #5=w20:dbl, element #6=w21:dbl, element #7=w22:dbl, element #8=w23:dbl)  [unwired: 8 in, 1 out]
        n29 = Bundle By Name(cluster=w24, "Delay increment"=w17, "Center Wavelength"=w18, "Frog Error was"=w19, "Temporal FWHM"=w20, "Spectral FWHM"=w21, "FWHM Time-Bandwidth Product"=w22, "RMS Time-Bandwidth Product"=w23) -> (w16:T1)
      }
      n30 = Array Max & Min(array=w12) -> (max value=→"max value (ms)":u32, max index (indices)=→"index":i32)  [unwired: 2 out]
    }
    frame True {
      w200 = T1 {"Delay increment"=0.0, "Center Wavelength"=0.0, "Frog Error was"=0.0, "Temporal FWHM"=0.0, "Spectral FWHM"=0.0, "FWHM Time-Bandwidth Product"=0.0, "RMS Time-Bandwidth Product"=0.0}  # FROG Cluster
      w204 = errorcluster {"status"=FALSE, "code"=0, "source"=""}  # error constant
      n31 = Index Array(array=T1[] [{"Delay increment"=36.8, "Center Wavelength"=809.3, "Frog Error was"=0.0344, "Temporal FWHM"=100.0, "Spectral FWHM"=7.96, "FWHM Time-Bandwidth Product"=0.364, "RMS Time-Bandwidth Product"=0.85}, {"Delay increment"=36.8, "Center Wavelength"=809.3, "Frog Error was"=0.036, "Temporal FWHM"=98.9, "Spectral FWHM"=9.04, "FWHM Time-Bandwidth Product"=0.408, "RMS Time-Bandwidth Product"=0.858}] ("FROG data")) -> (element=w203:T1)  [unwired: 1 in]
      n32 = Cluster To Array(cluster=w203) -> (array=w202:dbl[])
      n33 = for {
        tunnel: w202 -> [w208] mode=indexing
        tunnel: [w206] -> w199 mode=indexing
        n34 = Random Number (0-1)() -> (number: 0 to 1=w207:dbl)
        n35 = Increment(x=w207) -> (x+1=w205:dbl)
        n36 = Multiply(x=w208, y=w205) -> (x*y=w206:dbl)
      }
      n37 = Index Array(array=w199) -> (element #1=w198:dbl, element #2=w197:dbl, element #3=w196:dbl, element #4=w195:dbl, element #5=w194:dbl, element #6=w191:dbl, element #7=w190:dbl)  [unwired: 7 in]
      n38 = Bundle By Name(cluster=w200, "Delay increment"=w198, "Center Wavelength"=w197, "Frog Error was"=w196, "Temporal FWHM"=w195, "Spectral FWHM"=w194, "FWHM Time-Bandwidth Product"=w191, "RMS Time-Bandwidth Product"=w190) -> (w192:T1)
      n39 = Build Array(w192) -> (w193:T1[])
    }
  }
  "FROG data" <- w4
  "error out" <- w3
  "ExpFrog" <- w1
